vi "CAlex2_SetLegDH.vi"(8 "error in (no error)":errorcluster, 9 "End Effector Pos":T1={"Coord4"=[0.0, 0.0, 0.0, 1.0], "ID"=4}, 10 "ArmProperty":T2, 11 "CAlex2 in":refnum<class "CAlex2.lvclass">) -> (0 "error out":errorcluster, 3 "CAlex2 out":refnum<class "CAlex2.lvclass">)   [LabVIEW 2015, in "CAlex2.lvclass"]
uses:
  CAlex2.lvclass
  TypeDef/LowerBodyDim.ctl
  Body/PointOnBody.ctl
  Body/xyzO.ctl
  Body/Bodies.lvclass
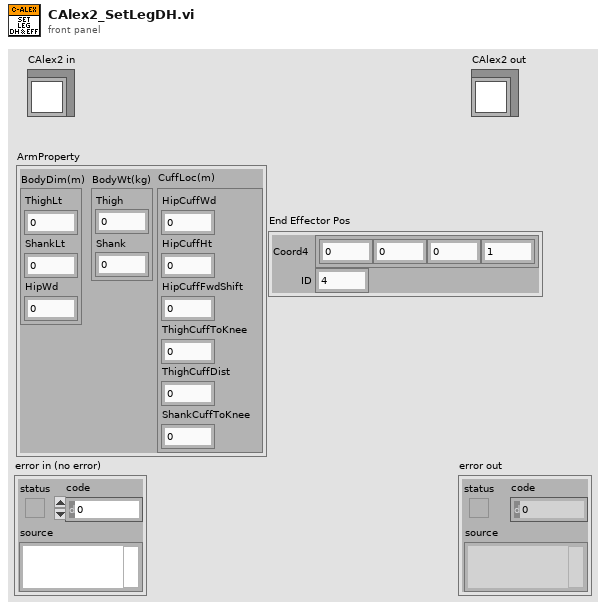
[diagram p1: front panel]
types:
  T1 = typedef "Bodies.lvclass/PointOnBody.ctl" = cluster{"Coord4":dbl[], "ID":i32}
  T2 = typedef "CAlex2.lvclass/LowerBodyDim.ctl" = cluster{"BodyDim(m)":cluster{"ThighLt":dbl, "ShankLt":dbl, "HipWd":dbl}, "BodyWt(kg)":cluster{"Thigh":dbl, "Shank":dbl}, "CuffLoc(m)":cluster{"HipCuffWd":dbl, "HipCuffHt":dbl, "HipCuffFwdShift":dbl, "ThighCuffToKnee":dbl, "ThighCuffDist":dbl, "ShankCuffToKnee":dbl}}
  T3 = typedef "Bodies.lvclass/xyzO.ctl" = enum16{"X", "Y", "Z", "O"}
  T4 = typedef "Bodies.lvclass/DH_parameters.ctl" = cluster{"unknown":enum16{"Theta", "Alpha", "a", "d"}, "a":dbl, "d":dbl, "alpha":dbl, "theta":dbl}
  T5 = cluster{"DH_parameters 2":T4, "CoM_Pos":T1, "Mass(kg)":dbl}
  T6 = cluster{"DH_parameters 2":T4, "CoM_Pos":T1, "Mass(kg)":dbl}[]
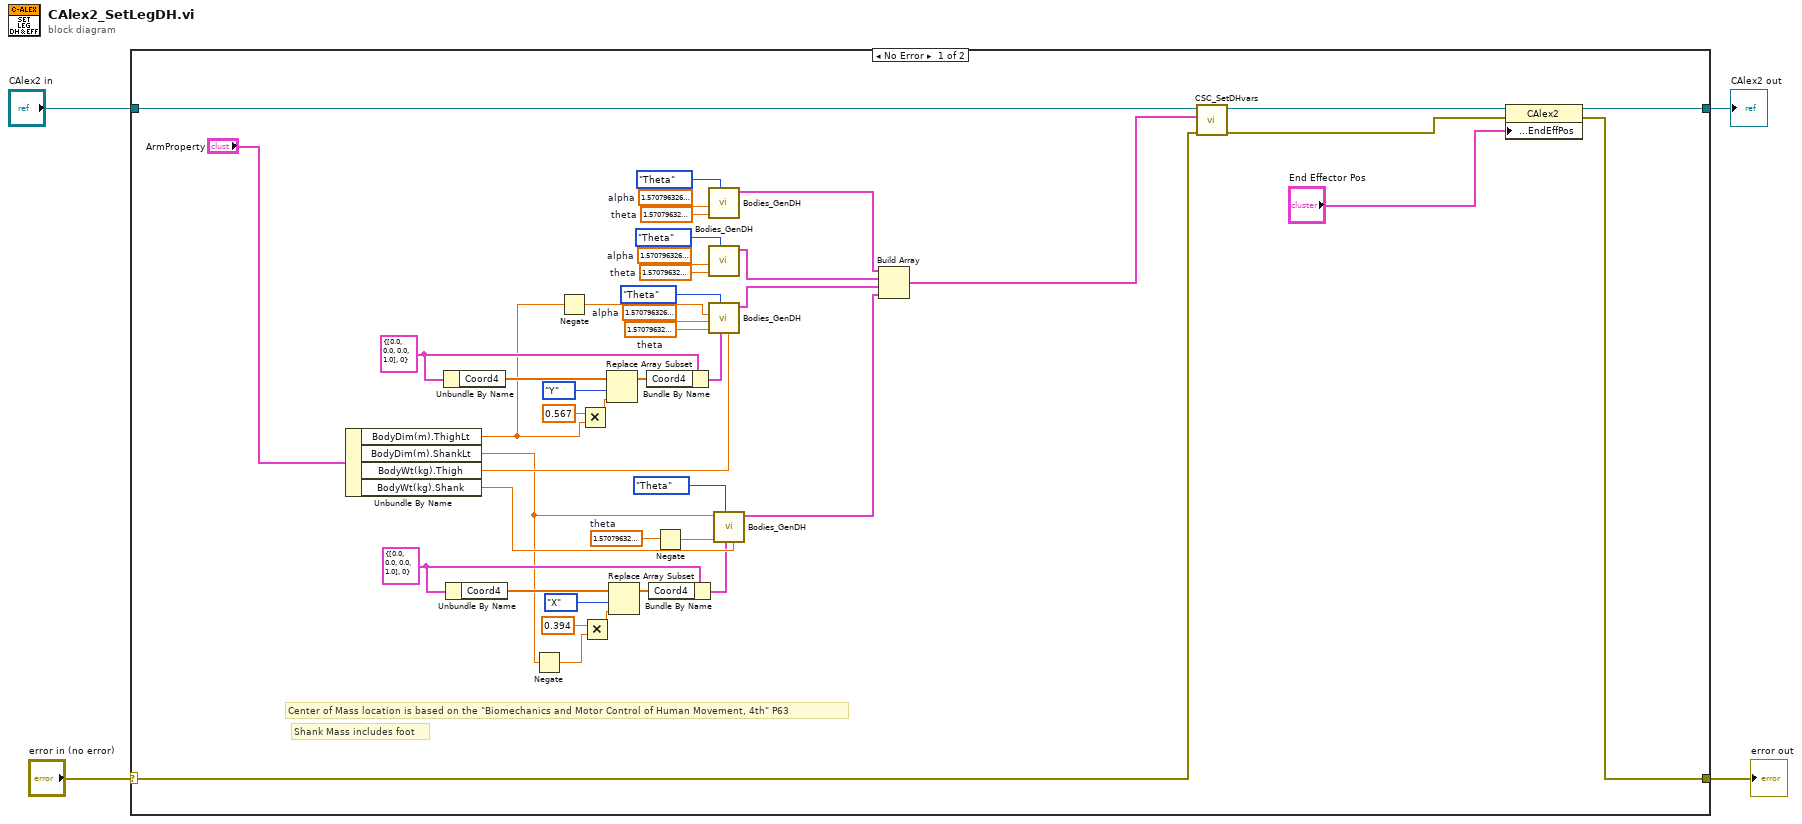
[diagram p0: block diagram]
diagram:
  n1 = case shown="No Error" "error in (no error)" {
    selector: "error in (no error)" -> [w5 w51]
    tunnel: [w36 w51] -> w3
    tunnel: [w37 w50] -> w1
    tunnel: "CAlex2 in" -> [w7 w50]
    frame No Error {
      w13 = T1 {"Coord4"=[0.0, 0.0, 0.0, 1.0], "ID"=0} ("CoM_Pos")
      w23 = T1 {"Coord4"=[0.0, 0.0, 0.0, 1.0], "ID"=0} ("CoM_Pos")
      w31 = 1.5707963267948966  # theta
      w32 = 1.5707963267948966  # theta
      w33 = 1.5707963267948966  # theta
      w34 = 1.5707963267948966  # theta
      w48 = 1.5707963267948966  # alpha
      w38 = 1.5707963267948966  # alpha
      w49 = 1.5707963267948966  # alpha
      # "Shank Mass includes foot"
      # "Center of Mass location is based on the \"Biomechanics and Motor Control of Human Movement, 4th\" P63"
      n2 = Unbundle By Name("ArmProperty") -> ("BodyDim(m).ThighLt"=w15:dbl, "BodyDim(m).ShankLt"=w11:dbl, "BodyWt(kg).Thigh"=w29:dbl, "BodyWt(kg).Shank"=w28:dbl)
      n3 = Unbundle By Name(w23) -> ("Coord4"=w24:dbl[])
      n4 = Unbundle By Name(w13) -> ("Coord4"=w19:dbl[])
      n5 = Negate(x=w11) -> (-x=w10:dbl)
      n6 = Negate(x=w15) -> (-x=w14:dbl)
      n7 = Multiply(x=0.567, y=w15) -> (x*y=w25:dbl)
      n8 = Multiply(x=0.394, y=w10) -> (x*y=w18:dbl)
      n9 = Replace Array Subset(array=w24, new element=w25, index=xyzO."Y" ("XYZ")) -> (w22:dbl[])
      n10 = Replace Array Subset(array=w19, new element=w18, index=xyzO."X" ("XYZ")) -> (w20:dbl[])
      n11 = Bundle By Name(cluster=w23, "Coord4"=w22) -> (w21:T1)
      n12 = Bundle By Name(cluster=w13, "Coord4"=w20) -> (w12:T1)
      n13 = Negate(x=w31) -> (-x=w30:dbl)
      n14 = call "Bodies_GenDH.vi"("Unknown(theta)"=enum16{"Theta", "Alpha", "a", "d"}."Theta" ("Unknown(Theta)"), "theta(0)"=w34, "alpha(0)"=w49) -> ("cluster"=w43:T5)  [unwired: 8 in]
      n15 = call "Bodies_GenDH.vi"("Unknown(theta)"=enum16{"Theta", "Alpha", "a", "d"}."Theta" ("Unknown(Theta)"), "theta(0)"=w33, "alpha(0)"=w38) -> ("cluster"=w42:T5)  [unwired: 8 in]
      n16 = call "Bodies_GenDH.vi"("Mass(kg)"=w29, "CoM_Pos"=w21, "Unknown(theta)"=enum16{"Theta", "Alpha", "a", "d"}."Theta" ("Unknown(Theta)"), "theta(0)"=w32, "alpha(0)"=w48, "d(0)"=w14) -> ("cluster"=w41:T5)  [unwired: 5 in]
      n17 = call "Bodies_GenDH.vi"("Mass(kg)"=w28, "CoM_Pos"=w12, "Unknown(theta)"=enum16{"Theta", "Alpha", "a", "d"}."Theta" ("Unknown(Theta)"), "theta(0)"=w30, "a(0)"=w11) -> ("cluster"=w40:T5)  [unwired: 6 in]
      n18 = Build Array(w43, w42, w41, w40) -> (w39:T6)
      n19 = call-dynamic "CSC_SetDHvars.vi"("error in (no error)"=w5, "KnownDHVars"=w39, "CSC in"=w7) -> ("error out"=w8:errorcluster, "CSC out"=w9:refnum<class "CAlex2.lvclass">)  [unwired: 7 in]
      n20 = property class="CAlex2"(reference=w9, error in=w8, "PropertyNodes:EndEffPos"="End Effector Pos") -> (reference out=w37:refnum<class "CAlex2.lvclass">, error out=w36:errorcluster)
    }
    frame Error {
    }
  }
  "error out" <- w3
  "CAlex2 out" <- w1
